vi "FFTvi.vi"(9 "Time Delta":dbl, 10 "Voltage INPUT2":dbl[](array[numeric]), 11 "Voltage INPUT1":dbl[](array[numeric])) -> (3 "FFT":dynamicdata(graph))   [LabVIEW 2012]
uses:
  <vilib>/express/express analysis/Spectral/Block/exnSpectralBlock spectral measurements peak poly.vi
  <vilib>/express/express analysis/Spectral/Block/exnSpectralBlock spectral measurements peak DDT.vi
  <vilib>/express/express analysis/Spectral/XNode/ExpressSpectralMeasurementsBlockNode.xnode
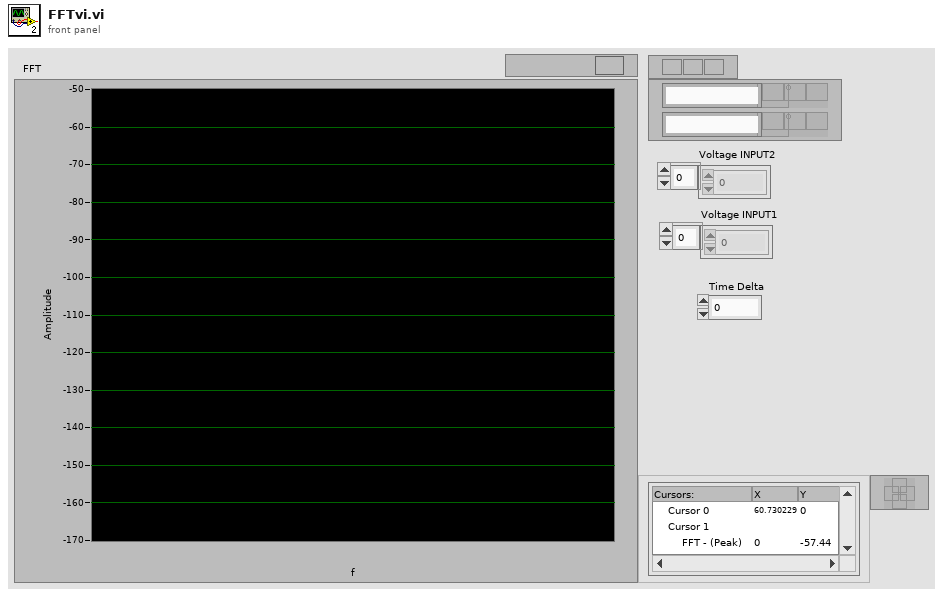
[diagram p1: front panel]
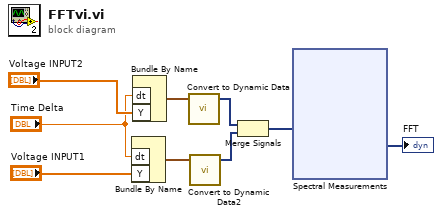
[diagram p0: block diagram]
diagram:
  n1 = Bundle By Name("dt"="Time Delta", "Y"="Voltage INPUT1") -> (w5:waveform(dbl))  [unwired: 1 in]
  n2 = Bundle By Name("dt"="Time Delta", "Y"="Voltage INPUT2") -> (w6:waveform(dbl))  [unwired: 1 in]
  n3 = call "Convert to Dynamic Data"("Array"=w6) -> ("Dynamic Data Type"=w9:dynamicdata)  [unwired: 3 in]
  n4 = call "Convert to Dynamic Data2"("Array"=w5) -> ("Dynamic Data Type"=w8:dynamicdata)  [unwired: 3 in]
  n5 = Merge Signals(w9, w8) -> (w4:dynamicdata)
  n6 = xnode "Spectral Measurements"("Signals"=w4) -> ("FFT - (Peak)"=→"FFT":dynamicdata)  [unwired: 1 in, 2 out]
